vi "Acquire S3DK.vi"(8 "error in (no error)":errorcluster, 10 "DATA IN":refnum<queue>, 11 "Hardware Resources in":T1={"State"=enum."Idle S3DK", "Settings"="", "S3DK"={"Signals"={"Phasor"=[], "Analog"=[], "Digital"=[]}}, "Tick"=0, "Online"=FALSE}) -> (0 "error out":errorcluster, 3 "Hardware Resources out":T1={"State"=enum."Idle S3DK", "Settings"="", "S3DK"={"Signals"={"Phasor"=[], "Analog"=[], "Digital"=[]}}, "Tick"=0, "Online"=FALSE})   [LabVIEW 2017, in "Acquisition.lvlib"]
doc: "Perform the acquisition. Replace the contents of this diagram with calls to acquisition hardware."
uses:
  Acquisition.lvlib
  Acquisition Settings.ctl
  Acquisition State.ctl
  support/libs/PMU Buffer/Buffer DATA cluster.ctl
  <vilib>/S3DK/PMU Recorder Light/PMU Recorder Light.lvlib
  support/libs/PMU Buffer/PMU data buffer.lvlib
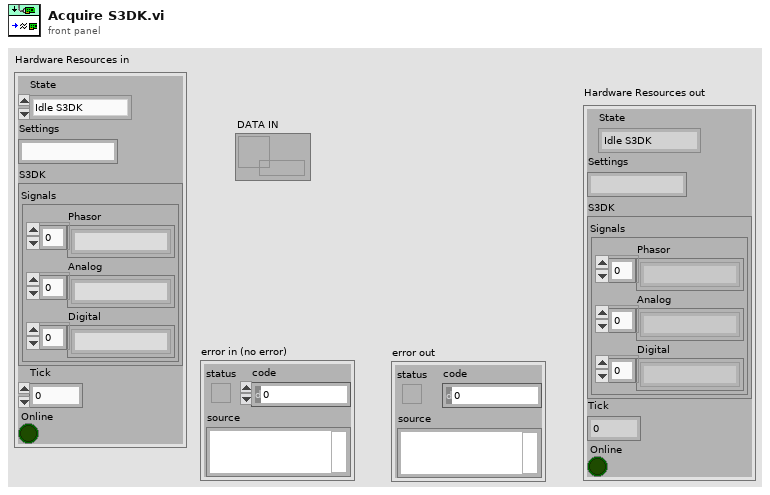
[diagram p1: front panel]
types:
  T1 = typedef "Acquisition.lvlib/Acquisition Settings.ctl" = cluster{"State":T2, "Settings":string, "S3DK":cluster{"Signals":cluster{"Phasor":string[], "Analog":string[], "Digital":string[]}}, "Tick":u32, "Online":bool}
  T2 = typedef "Acquisition.lvlib/Acquisition State.ctl" = enum16{"Idle", "Idle S3DK", "Acquiring S3DK", "Idle CSV", "Acquiring CSV"}
  T3 = typedef "PMU data buffer.lvlib/Buffer DATA cluster.ctl" = cluster{timestamp, csg[], sgl[]}
  T4 = cluster{timestamp, "Phasor Values":csg[], "Analog Values":sgl[]}
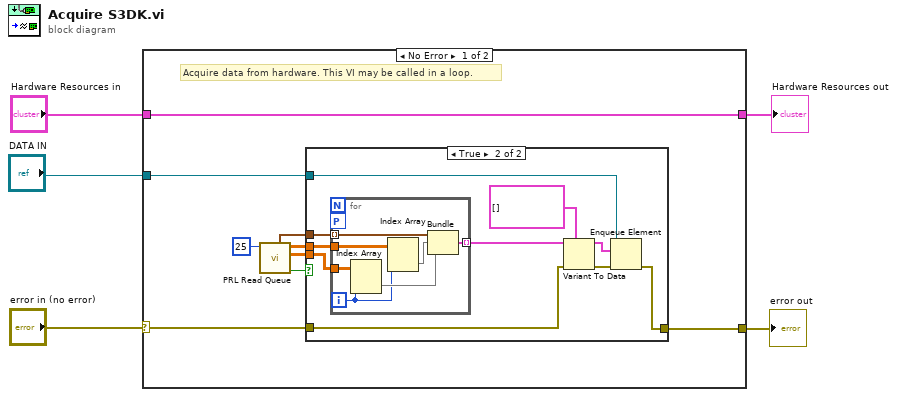
[diagram p0: block diagram]
diagram:
  # "Acquire data from hardware. This VI may be called in a loop."
  n1 = case shown="No Error" "error in (no error)" {
    selector: "error in (no error)" -> [w6 w32]
    tunnel: [w8 w32] -> w4
    tunnel: "Hardware Resources in" -> [w10 w33]
    tunnel: [w10 w33] -> w2
    tunnel: "DATA IN" -> [w14 _]
    frame No Error {
      n2 = call <vilib>:"PRL Read Queue.vi"("timeout in ms (5)"=25) -> ("Has Data?"=w7:bool, "Analog Values"=w11:sgl[][], "Phasor Values"=w12:csg[][], "Timestamp Values"=w13:timestamp[])  [unwired: 6 in, 1 out]
      n3 = case shown="True" w7 {
        tunnel: w14 -> [_ w24]
        tunnel: w13 -> [_ w23]
        tunnel: w12 -> [_ w22]
        tunnel: w11 -> [_ w21]
        tunnel: [_ w15] -> w8
        tunnel: w6 -> [_ w16]
        frame False {
        }
        frame True {
          n4 = for {
            tunnel: w23 -> [w31] mode=indexing
            tunnel: w22 -> [w29]
            tunnel: w21 -> [w28]
            tunnel: [w30] -> w19 mode=indexing
            workers-P: _ -> [_]
            i -> [w25]
            n5 = Index Array(array=w28, index (col)=w25) -> (element=w26:sgl[])  [unwired: 1 in]
            n6 = Index Array(array=w29, index (col)=w25) -> (element=w27:csg[])  [unwired: 1 in]
            n7 = Bundle(w31, "Phasor Values"=w27, "Analog Values"=w26) -> (w30:T4)  [unwired: 1 in]
          }
          n8 = Variant To Data(error in=w16, type=T3[] [], Variant=w19) -> (data=w18:T3[], error out=w17:errorcluster)
          n9 = Enqueue Element(queue=w24, element=w18, error in (no error)=w17) -> (error out=w15:errorcluster)  [unwired: 1 in, 2 out]
        }
      }
    }
    frame Error {
    }
  }
  "Hardware Resources out" <- w2
  "error out" <- w4
